vi "GetValue.vi"(8 "error in (no error)":errorcluster, 11 "node in":refnum<class "node.lvclass">) -> (0 "error out":errorcluster, 3 "node out":refnum<class "node.lvclass">)   [LabVIEW 2014, in "Linked List.lvlib" / "node.lvclass"]
uses:
  node.lvclass
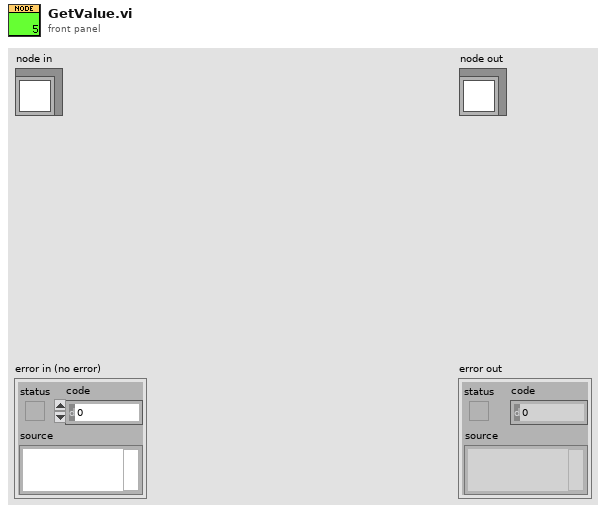
[diagram p1: front panel]
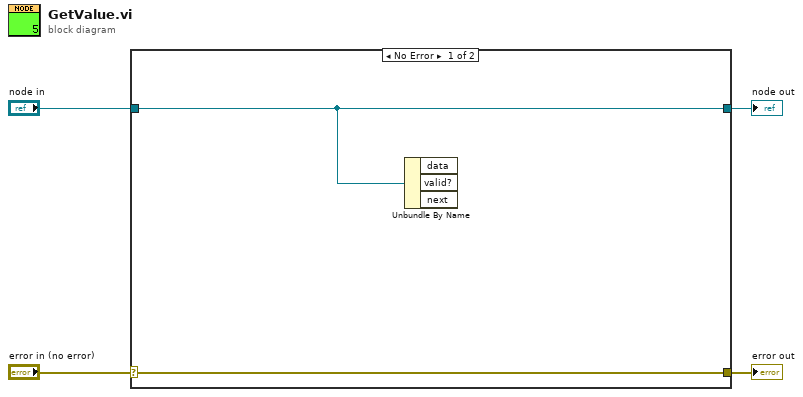
[diagram p0: block diagram]
diagram:
  n1 = case shown="No Error" "error in (no error)" {
    selector: "error in (no error)" -> [w6 w8]
    tunnel: [w6 w8] -> w3
    tunnel: [w5 w7] -> w1
    tunnel: "node in" -> [w5 w7]
    frame No Error {
      n2 = Unbundle By Name(w5) -> ()  [unwired: 3 out]
    }
    frame Error {
    }
  }
  "error out" <- w3
  "node out" <- w1
